vi "Clamp MAX_Simulaation.vi"(8 "error in (no error)":errorcluster, 10 "Image Type":T1 items=["Grayscale (U8)", "Grayscale (I16)", "Grayscale (SGL)", "Complex (CSG)", "RGB (U32)", "HSL (U32)", "RGB (U64)", "Grayscale (U16)"], 11 "Image Type 2":T1 items=["Grayscale (U8)", "Grayscale (I16)", "Grayscale (SGL)", "Complex (CSG)", "RGB (U32)", "HSL (U32)", "RGB (U64)", "Grayscale (U16)"]) -> (0 "error out":errorcluster, 3 "Refnum out":T2)   [LabVIEW 2019]
uses:
  <vilib>/vision/Image Controls.llb/IMAQ Image.ctl
  <vilib>/vision/NI_Vision_Development_Module.lvlib
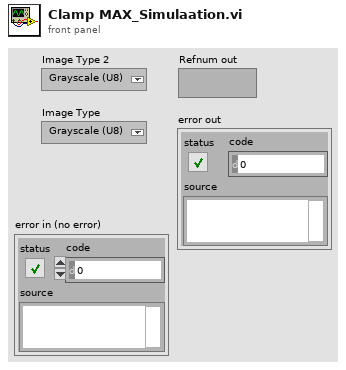
[diagram p1: front panel]
types:
  T1 = typedef "Image Type" = u32
  T2 = typedef "IMAQ Image.ctl" = refnum<image>
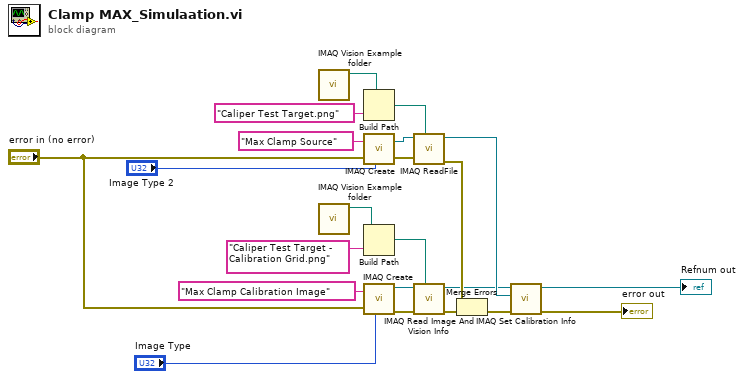
[diagram p0: block diagram]
diagram:
  n1 = call "IMAQ Vision Example folder.vi"() -> ("Example Image Path"=w13:path)  [unwired: 11 in]
  n2 = call "IMAQ Vision Example folder.vi"() -> ("Example Image Path"=w7:path)  [unwired: 11 in]
  n3 = Build Path(base path=w13, name or relative path="Caliper Test Target.png") -> (appended path=w14:path)
  n4 = call "IMAQ Create"("Image Name"="Max Clamp Source", "Image Type"="Image Type 2", "error in (no error)"="error in (no error)") -> ("New Image"=w11:T2, "error out"=w19:errorcluster)  [unwired: 1 in, 1 out]
  n5 = Build Path(base path=w7, name or relative path="Caliper Test Target - Calibration Grid.png") -> (appended path=w9:path)
  n6 = call "IMAQ Create"("Image Name"="Max Clamp Calibration Image", "Image Type"="Image Type", "error in (no error)"="error in (no error)") -> ("New Image"=w8:T2, "error out"=w18:errorcluster)  [unwired: 1 in, 1 out]
  n7 = call "IMAQ ReadFile"("File Path"=w14, "error in (no error)"=w19, "Image"=w11) -> ("error out"=w20:errorcluster, "Image Out"=w15:T2)  [unwired: 2 in, 5 out]
  n8 = call "IMAQ Read Image And Vision Info"("File Path"=w9, "error in (no error)"=w18, "Image"=w8) -> ("error out"=w21:errorcluster, "Image Out"=w10:T2)  [unwired: 1 in, 6 out]
  n9 = Merge Errors(w20, w21) -> (w22:errorcluster)
  n10 = call "IMAQ Set Calibration Info"("error in (no error)"=w22, "Image Dst"=w15, "Image Src"=w10) -> ("error out"=→"error out":errorcluster, "Calibrated Image"=→"Refnum out":T2)  [unwired: 1 in, 6 out]
